vi "Teleop.vi"(10 "Match Info":T1={"Autonomous Elapsed Seconds"=0.0, "TeleOp Elapsed Seconds"=0.0, "Disabled Elapsed Seconds"=0.0, "Visited Autonomous"=FALSE, "Visited TeleOp"=FALSE, "Visited Disabled"=FALSE, "Autonomous Settings"={"Autonomous Style"=enum."Independent", "VI Refnum"=refnum}}, 11 "Call Context":T2) -> ()   [LabVIEW 2011]
doc: "This VI is called for each TeleOp packet received from the DS where the robot is not disabled. It is often used to read from the joysticks and update I/O or to update setpoints for timed control loops. It should complete and return within 20 milliseconds or it may miss DS packets."
uses:
  <vilib>/Rock Robotics/WPI/DriverStation/WPI_DriverStationDerivedRobotMode.ctl
  <vilib>/Rock Robotics/WPI/DriverStation/WPI_DriverStationMatch Info.ctl
  Robot Global Data.vi
panel:
  out "Shifting Timer":u32
  out "Motor Set Timer":u32
  out "Default Code Timer":u32
  out "Shift Control":dbl=2.0 format="%.2f"
  in  "Left High":dbl=0.2
  in  "Right High":dbl=0.8
  in  "Left Mid":dbl=0.25
  in  "Right Mid":dbl=0.7
  in  "Shift Input 2":dbl
  in  "Left Low":dbl=0.8
  in  "Right Low":dbl=0.4
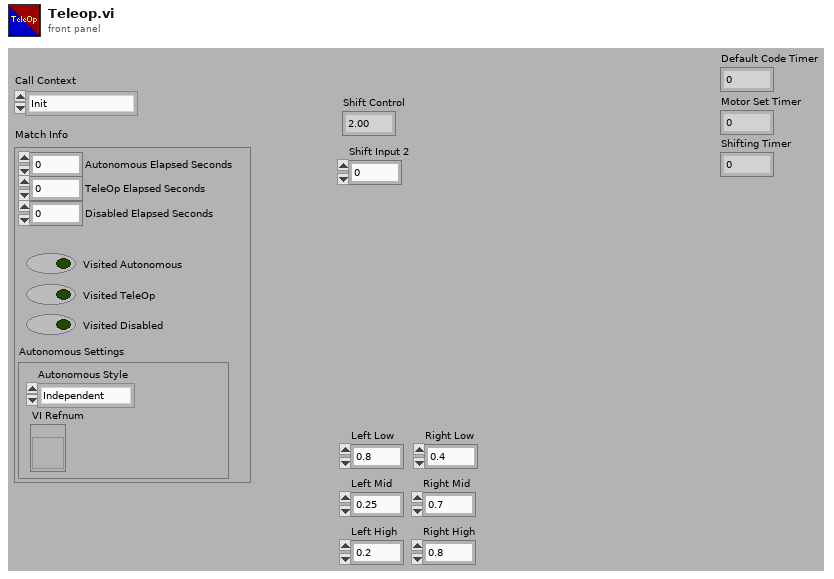
[diagram p1: front panel]
types:
  T1 = typedef "WPI_DriverStationMatch Info.ctl" = cluster{"Autonomous Elapsed Seconds":dbl, "TeleOp Elapsed Seconds":dbl, "Disabled Elapsed Seconds":dbl, "Visited Autonomous":bool, "Visited TeleOp":bool, "Visited Disabled":bool, "Autonomous Settings":cluster{"Autonomous Style":enum16{"Iterative", "Independent"}, "VI Refnum":refnum<vi>}}
  T2 = typedef "WPI_DriverStationDerivedRobotMode.ctl" = enum16{"Init", "Execute", "Stop"}
  T3 = typedef "WPI_JoystickDevRef.ctl" = cluster{"Device":T4}
  T4 = typedef "WPI_JoystickDeviceEnum.ctl" = enum16{"USB 1", "USB 2", "USB 3", "USB 4", "Kinect 1", "Kinect 2"}
  T5 = cluster{"axis 1 (x)":dbl, "axis 2 (y)":dbl, "axis 3 (throttle)":dbl, "axis 4":dbl, "axis 5":dbl, "axis 6":dbl}
  T6 = typedef "WPI_MotorControlDeviceRef.ctl" = cluster{"DeviceStatus":errorcluster, "Type":enum16{"PWM", "CAN"}, "PWM":cluster{"Digital Module":T7, "PWM Channel":T8, "DeadBand":T9}, "CAN":cluster{"Device Number":u8, "Control Mode":T10, "Semaphore":T11, "Max Vout":dbl}, "Invert":bool, "TransformRef":T12, "InvTransformRef":T12}
  T7 = typedef "FPGA_TypedefDigitalModule.ctl" = enum16{"Digital Module 1", "Digital Module 2"}
  T8 = typedef "FPGA_DIOPWMChannel.ctl" = enum8{"PWM 1", "PWM 2", "PWM 3", "PWM 4", "PWM 5", "PWM 6", "PWM 7", "PWM 8", "PWM 9", "PWM 10", "Invalid"}
  T9 = typedef "WPI_PWMDeadband.ctl" = cluster{"Name":string, "maxPositivePwm":i32, "minPositivePwm":i32, "centerPwm":i32, "maxNegativePwm":i32, "minNegativePwm":i32, "angularRange":u16}
  T10 = typedef "WPI_CANJaguar_ControlMode.ctl" = enum8{"Percent VBus", "Current", "Speed", "Position", "Voltage"}
  T11 = typedef "Semaphore RefNum" = refnum<k1>
  T12 = typedef "WPI_PWMTransform_ConPane.ctl" = refnum<vi>
  T13 = typedef "WPI_ServoDeviceRef.ctl" = cluster{"DeviceStatus":errorcluster, "Digital Module":T7, "PWM Channel":T8, "DeadBand":T9}
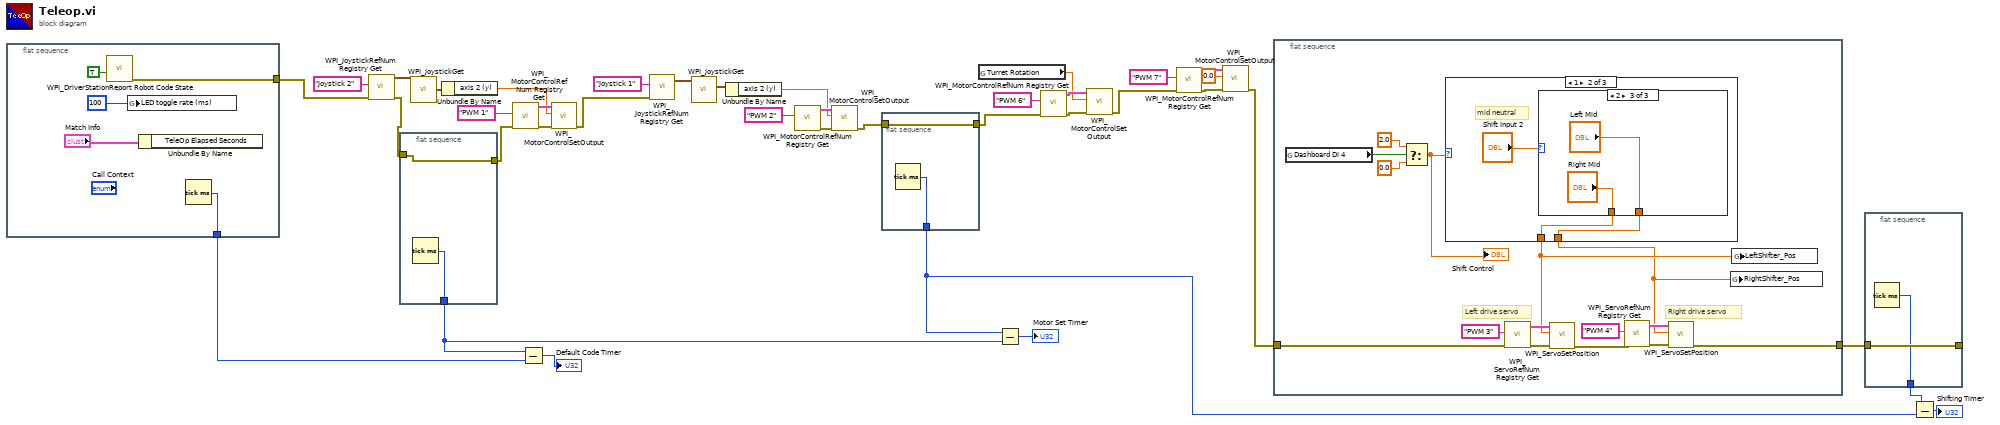
[diagram p0: block diagram]
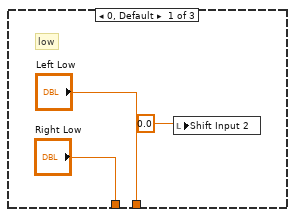
[diagram p2: hidden frame]
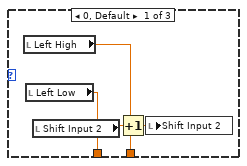
[diagram p3: hidden frame]
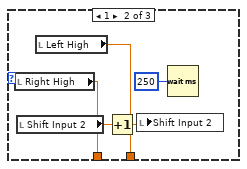
[diagram p4: hidden frame]
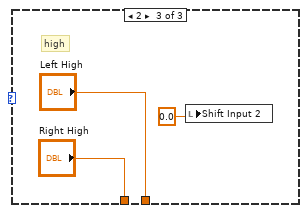
[diagram p5: hidden frame]
diagram:
  n1 = flat-sequence {
    tunnel: [w40] -> w13
    tunnel: [w39] -> w8
    frame #0 {
      n2 = call <vilib>:"WPI_DriverStationReport Robot Code State.vi"("TeleOp"=TRUE ("Autonomous")) -> ("error out"=w40:errorcluster)  [unwired: 10 in]
      n3 = global write "Robot Global Data.vi" "LED toggle rate (ms)"(u32 100 ("LED ms toggle rate")) -> ()
      n4 = Unbundle By Name("Match Info") -> ()  [unwired: 1 out]
      n5 = Tick Count (ms)() -> (millisecond timer value=w39:u32)
    }
  }
  n6 = call <vilib>:"WPI_JoystickRefNum Registry Get.vi"("error in (no error)"=w13, "refnum name"="Joystick 2") -> ("error out"=w12:errorcluster, "JoystickDevRef"=w25:T3)  [unwired: 8 in]
  n7 = flat-sequence {
    tunnel: [w45] -> w11
    tunnel: w12 -> [w45]
    tunnel: [w44] -> w6
    frame #0 {
      n8 = Tick Count (ms)() -> (millisecond timer value=w44:u32)
    }
  }
  n9 = call <vilib>:"WPI_JoystickGet.vi"("JoystickDevRef"=w25) -> ("Axes"=w21:T5)  [unwired: 4 in, 2 out]
  n10 = Unbundle By Name(w21) -> ("axis 2 (y)"=w23:dbl)
  n11 = call <vilib>:"WPI_MotorControlRefNum Registry Get.vi"("error in (no error)"=w11, "refnum name"="PWM 1") -> ("error out"=w35:errorcluster, "MotorControlDevRef"=w36:T6)  [unwired: 8 in]
  n12 = Subtract(x=w6, y=w8) -> (x-y=→"Default Code Timer":u32)
  n13 = call <vilib>:"WPI_MotorControlSetOutput.vi"("error in (no error)"=w35, "Output"=w23, "MotorControlDevRef"=w36) -> ("error out"=w16:errorcluster)  [unwired: 7 in, 1 out]
  n14 = call <vilib>:"WPI_JoystickRefNum Registry Get.vi"("error in (no error)"=w16, "refnum name"="Joystick 1") -> ("JoystickDevRef"=w28:T3)  [unwired: 8 in, 1 out]
  n15 = call <vilib>:"WPI_JoystickGet.vi"("JoystickDevRef"=w28) -> ("Axes"=w24:T5)  [unwired: 4 in, 2 out]
  n16 = Unbundle By Name(w24) -> ("axis 2 (y)"=w22:dbl)
  n17 = call <vilib>:"WPI_MotorControlRefNum Registry Get.vi"("refnum name"="PWM 2") -> ("error out"=w33:errorcluster, "MotorControlDevRef"=w34:T6)  [unwired: 9 in]
  n18 = call <vilib>:"WPI_MotorControlSetOutput.vi"("error in (no error)"=w33, "Output"=w22, "MotorControlDevRef"=w34) -> ("error out"=w10:errorcluster)  [unwired: 7 in, 1 out]
  n19 = flat-sequence {
    tunnel: [w47] -> w9
    tunnel: w10 -> [w47]
    tunnel: [w46] -> w4
    frame #0 {
      n20 = Tick Count (ms)() -> (millisecond timer value=w46:u32)
    }
  }
  n21 = global read "Robot Global Data.vi" "Turret Rotation"() -> (w29:dbl)
  n22 = Subtract(x=w4, y=w6) -> (x-y=→"Motor Set Timer":u32)
  n23 = call <vilib>:"WPI_MotorControlRefNum Registry Get.vi"("error in (no error)"=w9, "refnum name"="PWM 6") -> ("error out"=w32:errorcluster, "MotorControlDevRef"=w31:T6)  [unwired: 8 in]
  n24 = call <vilib>:"WPI_MotorControlSetOutput.vi"("error in (no error)"=w32, "Output"=w29, "MotorControlDevRef"=w31) -> ("error out"=w15:errorcluster)  [unwired: 7 in, 1 out]
  n25 = call <vilib>:"WPI_MotorControlRefNum Registry Get.vi"("error in (no error)"=w15, "refnum name"="PWM 7") -> ("error out"=w18:errorcluster, "MotorControlDevRef"=w19:T6)  [unwired: 8 in]
  n26 = call <vilib>:"WPI_MotorControlSetOutput.vi"("error in (no error)"=w18, "Output"=0.0, "MotorControlDevRef"=w19) -> ("error out"=w14:errorcluster)  [unwired: 7 in, 1 out]
  n27 = flat-sequence {
    tunnel: w14 -> [w52]
    tunnel: [w48] -> w2
    frame #0 {
      # "Right drive servo"
      # "Left drive servo"
      n28 = global read "Robot Global Data.vi" "Dashboard DI 4"() -> (w55:bool)
      n29 = Select(t=2.0, s=w55, f=0.0) -> (s? t:f=w57:dbl)
      "Shift Control" <- w57
      n30 = case shown="1" w57 {
        tunnel: ["Left Low" w67 "Left High"] -> w53
        tunnel: ["Right Low" w66 "Right High"] -> w54
        frame 0, Default {
          # "low"
          n31 = local write "Shift Input 2"(0.0 ("Input 2")) -> ()
        }
        frame 1 {
          # "mid neutral"
          n32 = case shown="2" "Shift Input 2" {
            tunnel: [w72 w73 "Left Mid"] -> w67
            tunnel: [w71 w74 "Right Mid"] -> w66
            frame 0, Default {
              n33 = local read "Left High"() -> (w72:dbl)
              n34 = local read "Left Low"() -> (w71:dbl)
              n35 = local read "Shift Input 2"() -> (w70:dbl)
              n36 = Increment(x=w70) -> (x+1=w69:dbl)
              n37 = local write "Shift Input 2"(w69) -> ()
            }
            frame 1 {
              n38 = local read "Right High"() -> (w74:dbl)
              n39 = local read "Shift Input 2"() -> (w76:dbl)
              n40 = local read "Left High"() -> (w73:dbl)
              n41 = Increment(x=w76) -> (x+1=w75:dbl)
              n42 = local write "Shift Input 2"(w75) -> ()
              n43 = Wait (ms)(milliseconds to wait=u32 250) -> ()  [unwired: 1 out]
            }
            frame 2 {
            }
          }
        }
        frame 2 {
          # "high"
          n44 = local write "Shift Input 2"(0.0 ("Input 2")) -> ()
        }
      }
      n45 = call <vilib>:"WPI_ServoRefNum Registry Get.vi"("error in (no error)"=w52, "refnum name"="PWM 3") -> ("error out"=w51:errorcluster, "ServoDeviceRef"=w62:T13)  [unwired: 8 out]
      n46 = call <vilib>:"WPI_ServoSetPosition.vi"("error in (no error)"=w51, "Position"=w54, "ServoDeviceRef"=w62) -> ("error out"=w50:errorcluster)  [unwired: 8 out]
      n47 = call <vilib>:"WPI_ServoRefNum Registry Get.vi"("error in (no error)"=w50, "refnum name"="PWM 4") -> ("error out"=w49:errorcluster, "ServoDeviceRef"=w58:T13)  [unwired: 8 out]
      n48 = call <vilib>:"WPI_ServoSetPosition.vi"("error in (no error)"=w49, "Position"=w53, "ServoDeviceRef"=w58) -> ("error out"=w48:errorcluster)  [unwired: 8 out]
      n49 = global write "Robot Global Data.vi" "RightShifter_Pos"(w53) -> ()
      n50 = global write "Robot Global Data.vi" "LeftShifter_Pos"(w54) -> ()
    }
  }
  n51 = flat-sequence {
    tunnel: [w84] -> _
    tunnel: w2 -> [w84]
    tunnel: [w83] -> w1
    frame #0 {
      n52 = Tick Count (ms)() -> (millisecond timer value=w83:u32)
    }
  }
  n53 = Subtract(x=w1, y=w4) -> (x-y=→"Shifting Timer":u32)
